vi "FGV_GuideTree.vi"(7 "Action":T1, 8 "error in":errorcluster caption="错误输入（无错误）", 9 "Tree_original":string[][](array[string]), 10 "Tag":string, 11 "Tree*":refnum<vi>) -> (0 "error out":errorcluster caption="错误输出", 1 "Running？":bool, 2 "UIname":string, 3 "Tree* out":refnum<vi>)   [LabVIEW 2017]
uses:
  FV_GuideTree.ctl
panel:
  in  "Image Path":path
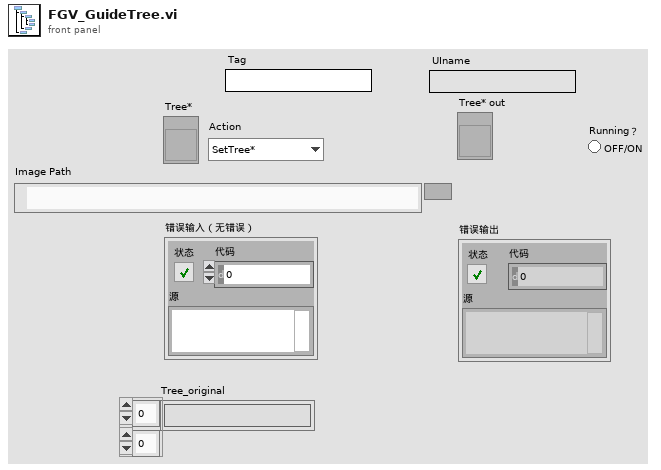
[diagram p1: front panel]
types:
  T1 = typedef "FV_GuideTree.ctl" = enum16{"SetTree*", "GetTree*", "InitlizeTree", "Get Item infor"}
  T2 = cluster{"Left Cell String":string, "Child Text":string[], "Child Tag":string, "Item Indent":i32, "Child Only?":bool, "Glyph Index":i32}
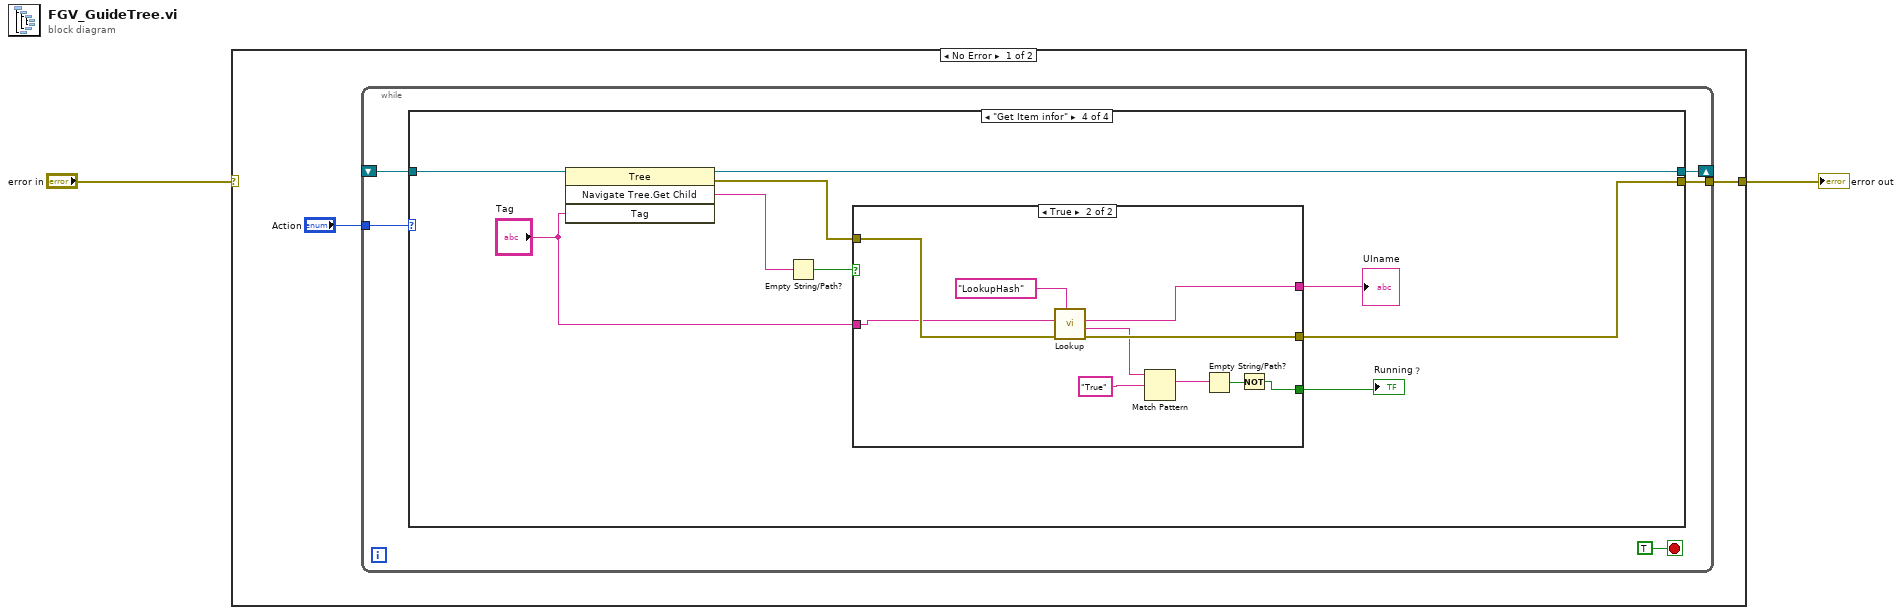
[diagram p0: block diagram]
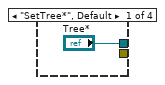
[diagram p2: hidden frame]
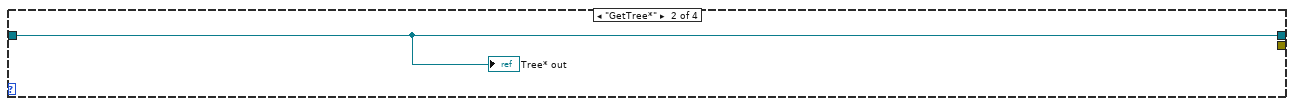
[diagram p3: hidden frame]
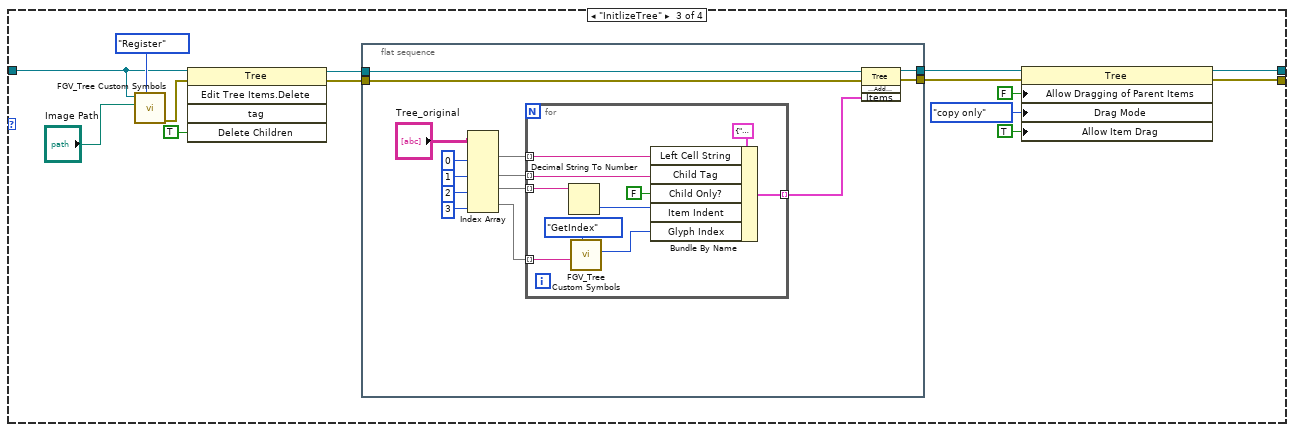
[diagram p4: hidden frame]
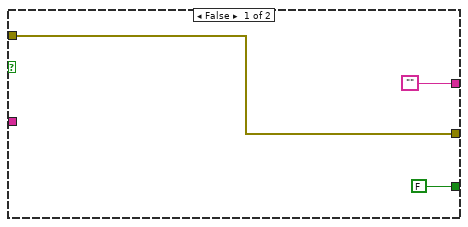
[diagram p5: hidden frame]
diagram:
  n1 = case shown="No Error" "error in" {
    selector: "error in" -> [_ w72]
    tunnel: [w3 w72] -> w2
    frame No Error {
      n2 = while {
        tunnel: "Action" -> [w8]
        shift-right: [w6] -> _
        shift-left: _ -> [w7]
        tunnel: [w5] -> w3
        stop <- TRUE stop-if-true
        n3 = case shown="\"Get Item infor\"" w8 {
          tunnel: w7 -> [_ w11 w20 w58]
          tunnel: ["Tree*" w11 w15 w57] -> w6
          tunnel: [_ _ w13 w50] -> w5
          frame "SetTree*", Default {
          }
          frame "GetTree*" {
            "Tree* out" <- w11
          }
          frame "InitlizeTree" {
            n4 = call "FGV_Tree Custom Symbols.vi"("Operation"=enum16{"Register", "GetIndex"}."Register", "Files"="Image Path", "tree refnum"=w20) -> ("error out"=w24:errorcluster)  [unwired: 7 in, 1 out]
            n5 = invoke class="Tree" method="Edit Tree Items.Delete"(reference=w20, error in=w24, "Delete Children"=TRUE ("删除子项？")) -> (reference out=w22:refnum<vi>, error out=w23:errorcluster)  [unwired: 2 in, 3 out]
            n6 = flat-sequence {
              tunnel: w23 -> [w39]
              tunnel: w22 -> [w38]
              tunnel: [w28] -> w16
              tunnel: [w27] -> w14
              frame #0 {
                n7 = Index Array(array="Tree_original", index (col) #1=0 ("禁用的索引 (列)"), index (col) #2=1 ("索引 (列)"), index (col) #3=2 ("索引 (列)"), index (col) #4=3 ("索引 (列)")) -> (element #1=w36:string[], element #2=w32:string[], element #3=w29:string[], element #4=w30:string[])  [unwired: 4 in]
                n8 = for {
                  tunnel: [w48] -> w34 mode=indexing
                  tunnel: w36 -> [w45] mode=indexing
                  tunnel: w30 -> [w44] mode=indexing
                  tunnel: w32 -> [w42] mode=indexing
                  tunnel: w29 -> [w41] mode=indexing
                  n9 = Decimal String To Number(string=w41) -> (number=w43:i32)  [unwired: 2 in, 1 out]
                  n10 = call "FGV_Tree Custom Symbols.vi"("Operation"=enum16{"Register", "GetIndex"}."GetIndex", "PicName"=w44) -> ("PicIndex"=w46:i32)  [unwired: 8 in, 1 out]
                  n11 = Bundle By Name(cluster=T2 {"Left Cell String"="", "Child Text"=[], "Child Tag"="", "Item Indent"=0, "Child Only?"=FALSE, "Glyph Index"=0} ("Item"), "Left Cell String"=w45, "Child Tag"=w42, "Child Only?"=FALSE, "Item Indent"=w43, "Glyph Index"=w46) -> (w48:T2)
                }
                n12 = invoke class="Tree" method="Edit Tree Items.Add Multiple Items to End"(reference=w38, error in=w39, "Items"=w34) -> (reference out=w28:refnum<vi>, error out=w27:errorcluster)  [unwired: 1 in, 2 out]
              }
            }
            n13 = property class="Tree"(reference=w16, error in=w14, "Allow Dragging of Parent Items"=FALSE ("拖曳/放置:允许拖曳父项"), "Drag Mode"=enum32{"copy or move", "copy only", "move only"}."copy only" ("拖曳/放置:拖曳模式"), "Allow Item Drag"=TRUE ("拖曳/放置:允许拖曳")) -> (reference out=w15:refnum<vi>, error out=w13:errorcluster)
          }
          frame "Get Item infor" {
            n14 = invoke class="Tree" method="Navigate Tree.Get Child"(reference=w58, "Tag"="Tag") -> (reference out=w57:refnum<vi>, error out=w51:errorcluster, "Navigate Tree:Get Child"=w56:string)  [unwired: 2 in, 1 out]
            n15 = Empty String/Path?(string/path=w56) -> (empty?=w55:bool)
            n16 = case shown="True" w55 {
              tunnel: "Tag" -> [_ w70]
              tunnel: ["" w69] -> w53
              tunnel: [FALSE w63] -> w52
              tunnel: w51 -> [w59 w71]
              tunnel: [w59 w68] -> w50
              frame False {
              }
              frame True {
                n17 = call "Lookup.vi"("Table"="LookupHash", "error in (no error)"=w71, "Tag"=w70) -> ("error out"=w68:errorcluster, "Item2"=w67:string, "Item1"=w69:string)  [unwired: 6 in]
                n18 = Match Pattern(string=w67, regular expression="True") -> (match substring=w65:string)  [unwired: 1 in, 3 out]
                n19 = Empty String/Path?(string/path=w65) -> (empty?=w64:bool)
                n20 = Not(x=w64) -> (.not. x?=w63:bool)
              }
            }
            "UIname" <- w53
            "Running？" <- w52
          }
        }
      }
    }
    frame Error {
    }
  }
  "error out" <- w2
